vi "IncrementDurabilityConditions.vi"(11 "Configuration Data in":T1) -> (2 "Boolean":bool, 3 "Configuration Data out":T1)   [LabVIEW 2026, in "Acquisition.lvlib"]
uses:
  Acquisition.lvlib
  controls/Test Config Data.ctl
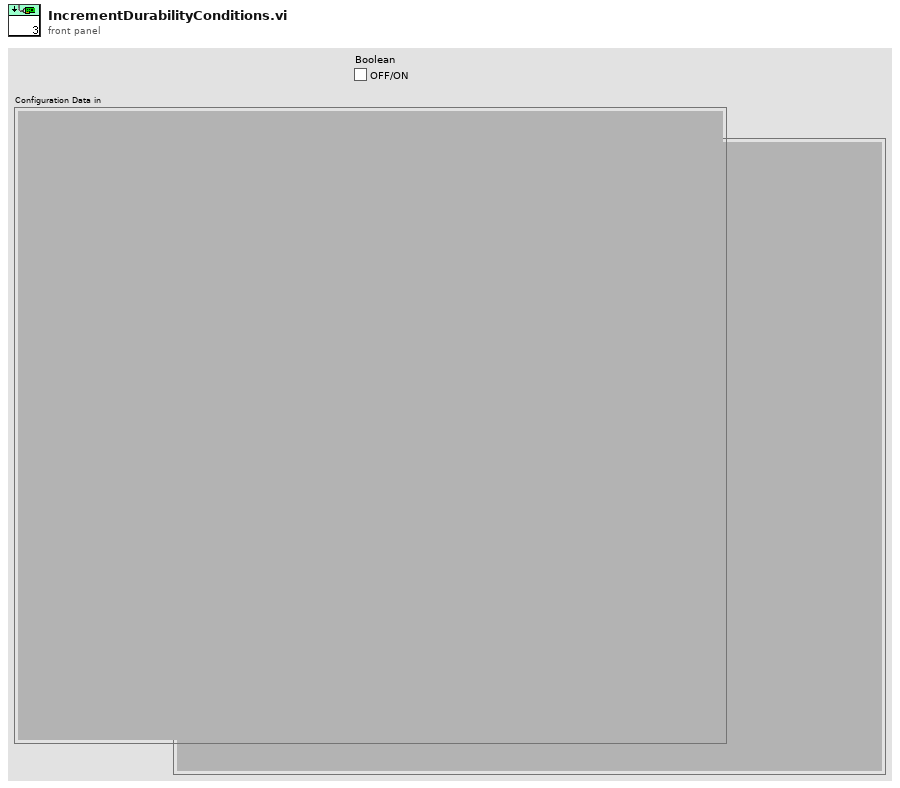
[diagram p1: front panel]
types:
  T1 = typedef "Test Config Data.ctl" = cluster{}
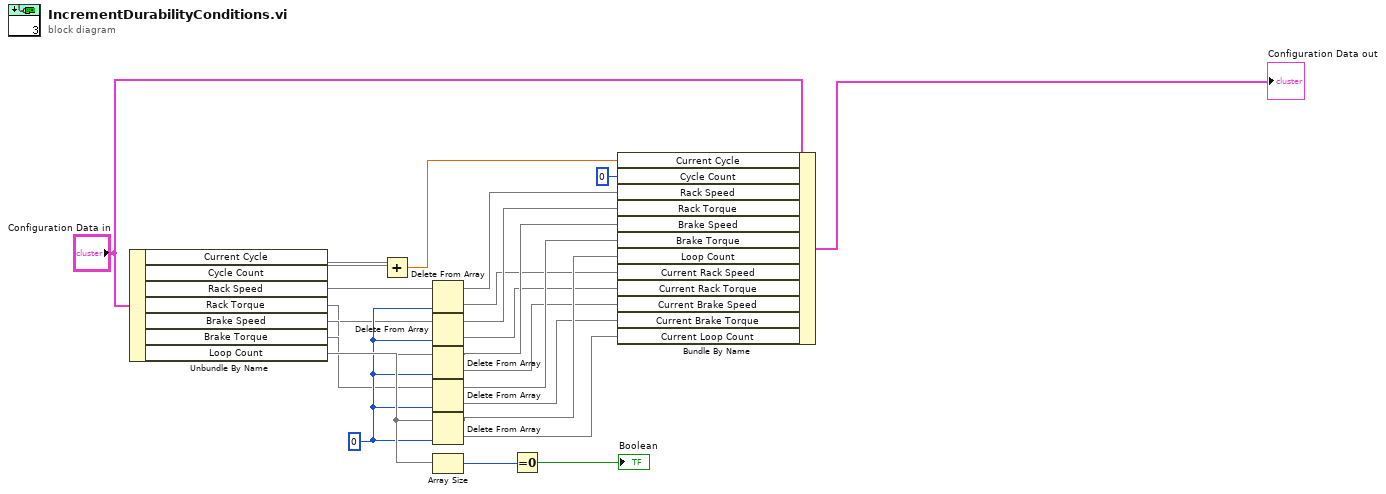
[diagram p0: block diagram]
diagram:
  w17 = 0 ("index")
  n1 = Unbundle By Name("Configuration Data in") -> ("Current Cycle"=w20, "Cycle Count"=w19, "Rack Speed"=w3, "Rack Torque"=w4, "Brake Speed"=w5, "Brake Torque"=w6, "Loop Count"=w22)
  n2 = Add(x=w20, y=w19) -> (x+y=w21:dbl)
  n3 = Delete From Array(array=w3, index=w17) -> (deleted portion=w7, array with subset deleted=w12)  [unwired: 1 in]
  n4 = Delete From Array(array=w4, index=w17) -> (deleted portion=w8, array with subset deleted=w13)  [unwired: 1 in]
  n5 = Delete From Array(array=w5, index=w17) -> (deleted portion=w9, array with subset deleted=w14)  [unwired: 1 in]
  n6 = Delete From Array(array=w6, index=w17) -> (deleted portion=w10, array with subset deleted=w15)  [unwired: 1 in]
  n7 = Delete From Array(array=w22, index=w17) -> (deleted portion=w11, array with subset deleted=w16)  [unwired: 1 in]
  n8 = Array Size(array=w22) -> (size(s)=w23:i32)
  n9 = Equal To 0?(x=w23) -> (x = 0?=→"Boolean":bool)
  n10 = Bundle By Name(cluster="Configuration Data in", "Current Cycle"=w21, "Cycle Count"=u64 0, "Rack Speed"=w12, "Rack Torque"=w13, "Brake Speed"=w14, "Brake Torque"=w15, "Loop Count"=w16, "Current Rack Speed"=w7, "Current Rack Torque"=w8, "Current Brake Speed"=w9, "Current Brake Torque"=w10, "Current Loop Count"=w11) -> (→"Configuration Data out":T1)
